vi "Boolean Latch.vi"(1 "Input":bool) -> (0 "Output":bool)   [LabVIEW 2015]
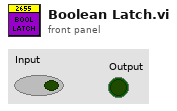
[diagram p1: front panel]
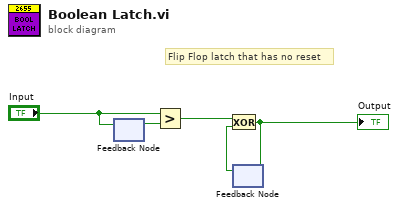
[diagram p0: block diagram]
diagram:
  # "Flip Flop latch that has no reset"
  n1 = feedback #1() -> (w3:bool)  [unwired: 1 in]
  n2 = feedback-in #1("Input") -> ()
  n3 = Greater?(x="Input", y=w3) -> (0:w4:bool)
  n4 = feedback #2() -> (w5:bool)  [unwired: 1 in]
  n5 = Exclusive Or(1:w5, 2:w4) -> (0:w1:bool)
  "Output" <- w1
  n6 = feedback-in #2(w1) -> ()
